vi "Sum3.vi"(2 "stream 3":T1, 3 "stream 2":T1, 4 "stream 1":T1) -> (0 "stream out":T1)   [LabVIEW 2023]
uses:
  <extravilib>/ChannelInstances/Stream-dbl/)Channel.ctl
  <extravilib>/ChannelInstances/Stream-dbl/Read With Abort.vi
  <extravilib>/ChannelInstances/Stream-dbl/Write With Abort.vi
  <extravilib>/ChannelInstances/Stream-dbl/EndpointRead.vi
  <extravilib>/ChannelInstances/Stream-dbl/Endpoint.vi
  <extravilib>/ChannelInstances/Stream-dbl/)Channel.vi
  <resource>/ChannelSupport/_ChannelSupport/WaitIfNeeded.vi
  <extravilib>/ChannelInstances/Stream-dbl.lvlib
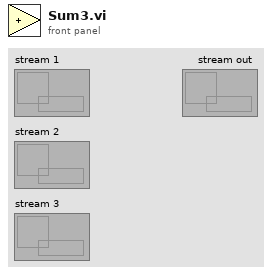
[diagram p1: front panel]
types:
  T1 = typedef "Stream-dbl.lvlib/)Channel.ctl" = refnum<queue>
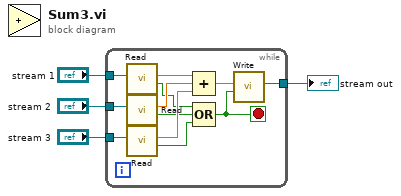
[diagram p0: block diagram]
diagram:
  n1 = while {
    tunnel: [w6] -> w3
    tunnel: "stream 1" -> [w16]
    tunnel: "stream 2" -> [w15]
    tunnel: "stream 3" -> [w14]
    stop <- w5 stop-if-true
    n2 = call <extravilib>:"Read.vi"("channel"=w16) -> ("last element?"=w8:bool, "element"=w13:dbl)  [unwired: 6 in, 3 out]
    n3 = call <extravilib>:"Read.vi"("channel"=w15) -> ("last element?"=w9:bool, "element"=w12:dbl)  [unwired: 6 in, 3 out]
    n4 = call <extravilib>:"Read.vi"("channel"=w14) -> ("last element?"=w10:bool, "element"=w11:dbl)  [unwired: 6 in, 3 out]
    n5 = Compound Arithmetic op=ADD(w13, w12, w11) -> (w7:dbl)
    n6 = Compound Arithmetic op=OR(w8, w9, w10) -> (w5:bool)
    n7 = call <extravilib>:"Write.vi"("last element? (F)"=w5, "element"=w7) -> ("channel"=w6:T1)  [unwired: 7 in, 2 out]
  }
  "stream out" <- w3
